vi "Configure DisLevel Core.vi"(8 "error in (no error)":errorcluster, 10 "DiscLvl":dbl[unit], 11 "CS++MCS in":refnum<class "CS++MCS.lvclass">) -> (0 "error out":errorcluster, 3 "CS++MCS out":refnum<class "CS++MCS.lvclass">)   [LabVIEW 2016, in "CS++MCS.lvlib" / "CS++MCS.lvclass"]
doc: "This VI configures the Level used for discriminating analog event signals."
uses:
  CS++MCS.lvclass
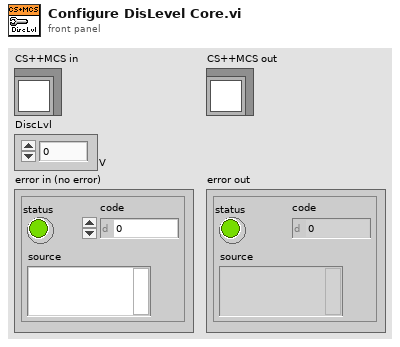
[diagram p1: front panel]
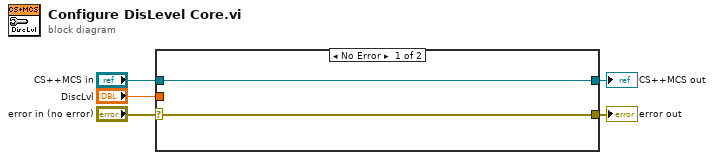
[diagram p0: block diagram]
diagram:
  n1 = case shown="No Error" "error in (no error)" {
    selector: "error in (no error)" -> [w6 w9]
    tunnel: [w6 w9] -> w4
    tunnel: [w7 w8] -> w2
    tunnel: "CS++MCS in" -> [w7 w8]
    tunnel: "DiscLvl" -> [_ _]
    frame No Error {
    }
    frame Error {
    }
  }
  "error out" <- w4
  "CS++MCS out" <- w2
